vi "Open Form.vi"(8 "error in (no error)":errorcluster, 10 "Panel Form Controller":refnum<class "Panel Form Controller.lvclass">, 11 "Form Model Messages in":refnum<class "Form Model Messages.lvclass">) -> (0 "error out":errorcluster, 3 "Form Model Messages out":refnum<class "Form Model Messages.lvclass">)   [LabVIEW 2020, in "Form Model Interfaces.lvlib" / "Form Model Messages.lvclass"]
uses:
  Form Model Messages/Form Model Messages.lvclass
  Forms Controller/Form Controller/Panel Form Controller.lvclass
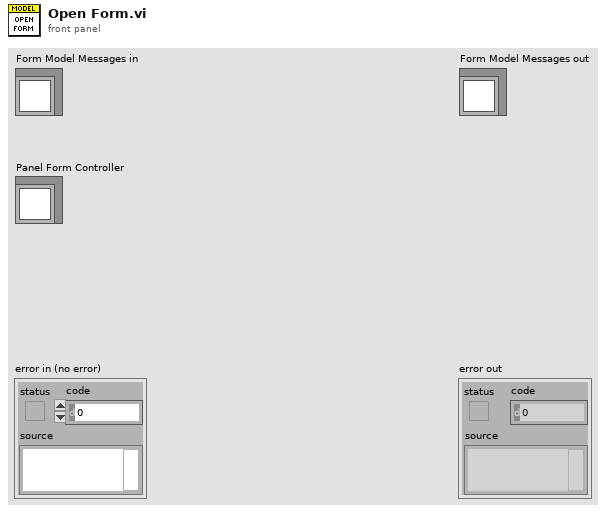
[diagram p1: front panel]
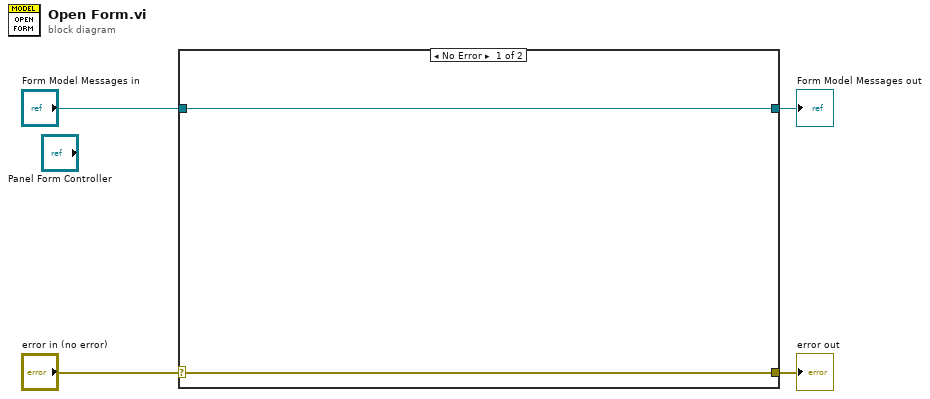
[diagram p0: block diagram]
diagram:
  n1 = case shown="No Error" "error in (no error)" {
    selector: "error in (no error)" -> [w6 w8]
    tunnel: [w6 w8] -> w3
    tunnel: [w5 w7] -> w1
    tunnel: "Form Model Messages in" -> [w5 w7]
    frame No Error {
    }
    frame Error {
    }
  }
  "error out" <- w3
  "Form Model Messages out" <- w1
